vi "close COM port.vi"() -> ()   [LabVIEW 2017]
uses:
  <instrlib>/Harvard Apparatus PHD Ultra Series/Harvard Apparatus PHD Ultra Series.lvlib
panel:
  in  "VISA resource name 4":refnum<visa-resource-name>="COM4"
  in  "VISA resource name 3":refnum<visa-resource-name>="COM12"
  in  "VISA resource name 2":refnum<visa-resource-name>="COM9"
  in  "VISA resource name":refnum<visa-resource-name>="COM11"
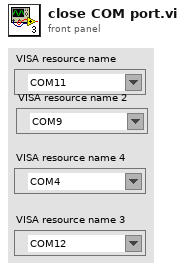
[diagram p1: front panel]
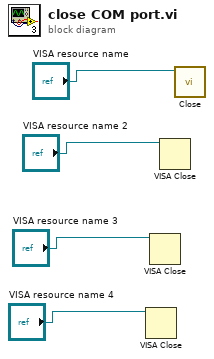
[diagram p0: block diagram]
diagram:
  n1 = VISA Close(VISA resource name="VISA resource name 4") -> ()  [unwired: 1 in, 1 out]
  n2 = VISA Close(VISA resource name="VISA resource name 3") -> ()  [unwired: 1 in, 1 out]
  n3 = VISA Close(VISA resource name="VISA resource name 2") -> ()  [unwired: 1 in, 1 out]
  n4 = call <instrlib>:"Close.vi"("VISA resource name"="VISA resource name") -> ()  [unwired: 10 in, 1 out]
